vi "PhysMon-Options Dialog.vi"(0 "Options":T1={"Min Interval"=0.0, "HR from ABR?"=FALSE, "HR Scale"={"Slope"=0.0, "Offset"=0.0, "Limits"={"Min"=0.0, "Max"=0.0}, "term config"=-1}, "Temp Scale"={"Slope"=0.0, "Offset"=0.0, "Limits"={"Min"=0.0, "Max"=0.0}, "term config"=-1}, "Lock?"=FALSE, "Temp Sensor"=enum."YSI", "EKG"={"Sample duration (s)"=0.0}} {"Temp Scale"."term config" items=["default"=-1, "RSE"=10083, "NRSE"=10078, "Differential"=10106, "Pseudodifferential"=12529]; "HR Scale"."term config" items=["default"=-1, "RSE"=10083, "NRSE"=10078, "Differential"=10106, "Pseudodifferential"=12529]}) -> (4 "Options Out":T1={"Min Interval"=0.0, "HR from ABR?"=FALSE, "HR Scale"={"Slope"=0.0, "Offset"=0.0, "Limits"={"Min"=0.0, "Max"=0.0}, "term config"=-1}, "Temp Scale"={"Slope"=0.0, "Offset"=0.0, "Limits"={"Min"=0.0, "Max"=0.0}, "term config"=-1}, "Lock?"=FALSE, "Temp Sensor"=enum."YSI", "EKG"={"Sample duration (s)"=0.0}} {"Temp Scale"."term config" items=["default"=-1, "RSE"=10083, "NRSE"=10078, "Differential"=10106, "Pseudodifferential"=12529]; "HR Scale"."term config" items=["default"=-1, "RSE"=10083, "NRSE"=10078, "Differential"=10106, "Pseudodifferential"=12529]}, 8 "Canceled?":bool)   [LabVIEW 2020]
uses:
  Typedefs/PhysMon-Options.ctl
  Typedefs/PhysMon-Scale.ctl
  Typedefs/PhysMon-TempSensor.ctl
  Typedefs/PhysMon-HR From EKG Settings.ctl
panel:
  in  "HRTab":enum32{"Cardiotach", "EKG"}(tab)
  in  "HR Slope":dbl caption="Scale (bpm/V)"
  in  "HR Offset":dbl caption="Offset (bpm)"
  in  "Reset HR":bool
  in  "Test":bool
  in  "Sample size (s)":dbl
  in  "Sensor":enum16{"YSI", "FHC", "Custom"}(ring)
  in  "dummy":i32(ring)=10078 items=["default"=-1, "RSE"=10083, "NRSE"=10078, "Differential"=10106, "Pseudodifferential"=12529]
  in  "Calibrate":bool
  in  "TInputConfig":i32(ring) caption="Input configuration" items=["default"=-1, "RSE"=10083, "NRSE"=10078, "Differential"=10106, "Pseudodifferential"=12529]
  in  "Lock?":bool caption="Acquire vitals only when the system is idle"
  in  "HR from ABR":bool caption="Measure from raw EKG"
  in  "Reset Temp":bool
  in  "Temp Offset":dbl caption="Offset (deg C)"
  in  "Temp Slope":dbl caption="Scale (deg C/V)"
  in  "HR Max":dbl caption="Alarm max (bpm)"
  in  "HR Min":dbl caption="Alarm min (bpm)"
  in  "Min Interval":dbl caption="Minimum time between vital signs acquisition (min)"
  in  "Cancel":bool
  in  "OK":bool
  # "Heart Rate"
  # "Temperature"
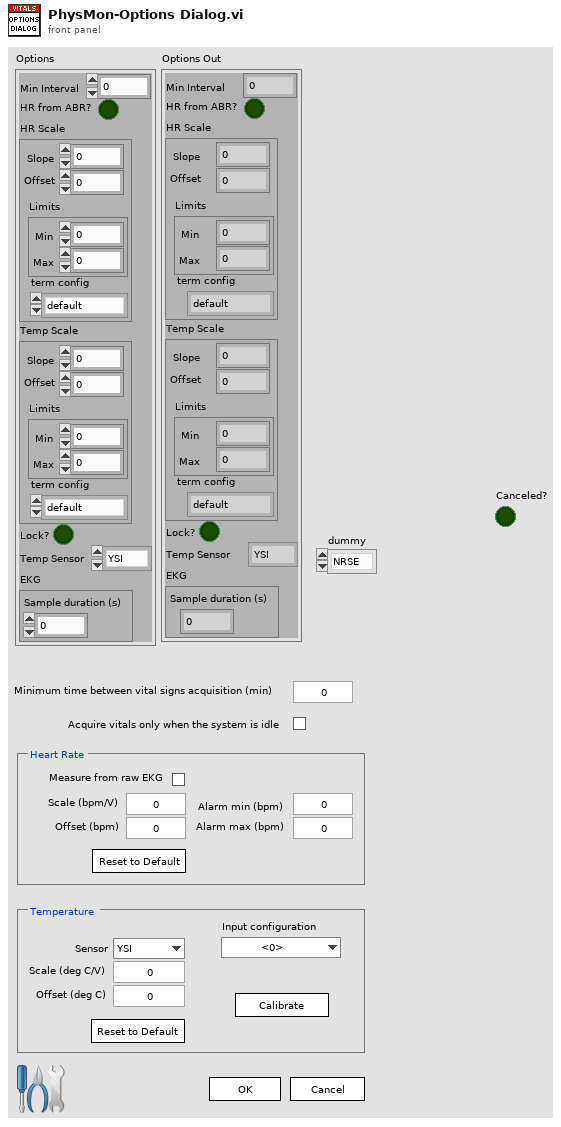
[diagram p1: front panel]
types:
  T1 = typedef "PhysMon-Options.ctl" = cluster{"Min Interval":dbl, "HR from ABR?":bool, "HR Scale":T2, "Temp Scale":T2, "Lock?":bool, "Temp Sensor":T3, "EKG":T4}
  T2 = typedef "PhysMon-Scale.ctl" = cluster{"Slope":dbl, "Offset":dbl, "Limits":cluster{"Min":dbl, "Max":dbl}, "term config":i32}
  T3 = typedef "PhysMon-TempSensor.ctl" = enum16{"YSI", "FHC", "Custom"}
  T4 = typedef "PhysMon-HR From EKG Settings.ctl" = cluster{"Sample duration (s)":dbl}
  T5 = enum8{"Enabled", "Disabled", "Disabled and Grayed Out"}
  T6 = typedef "LVStringsAndValuesArrayTypeDef_I32.ctl" = cluster{"String":string, "Value":i32}[]
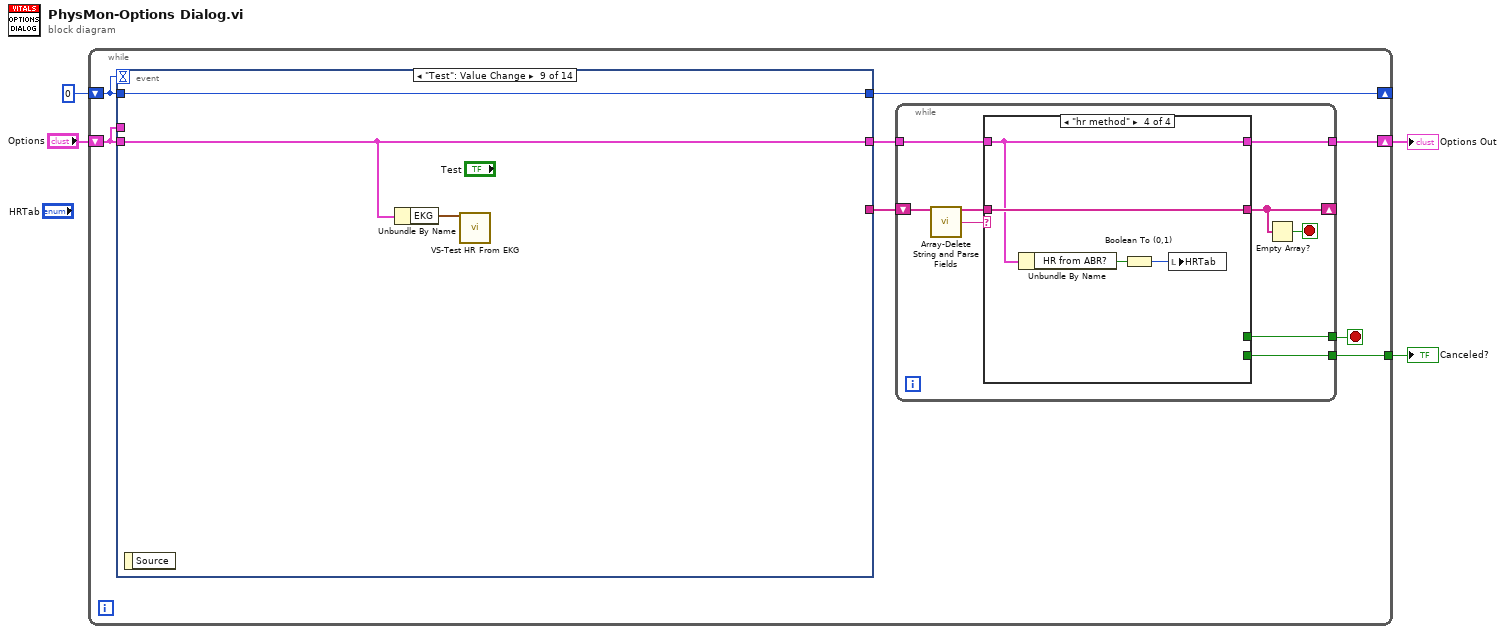
[diagram p0: block diagram]
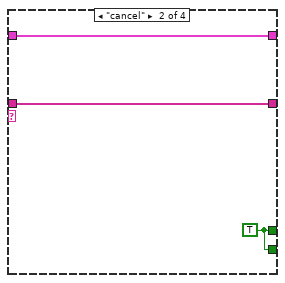
[diagram p3: hidden frame]
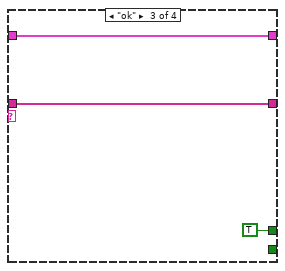
[diagram p4: hidden frame]
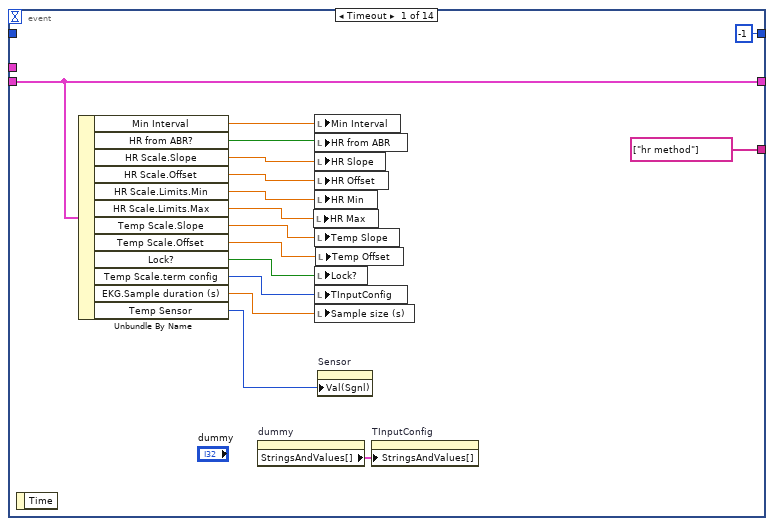
[diagram p5: hidden frame]
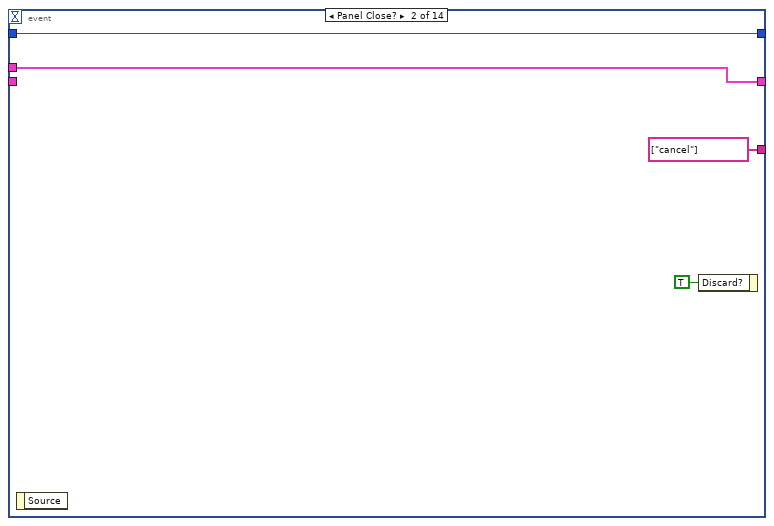
[diagram p6: hidden frame]
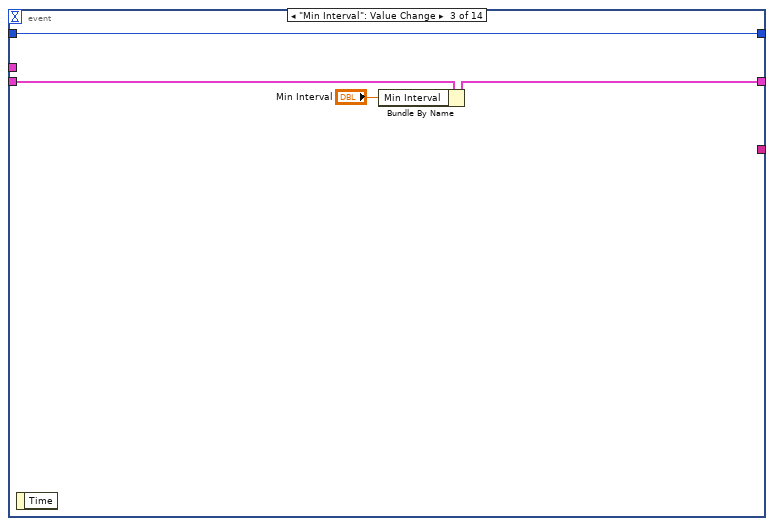
[diagram p7: hidden frame]
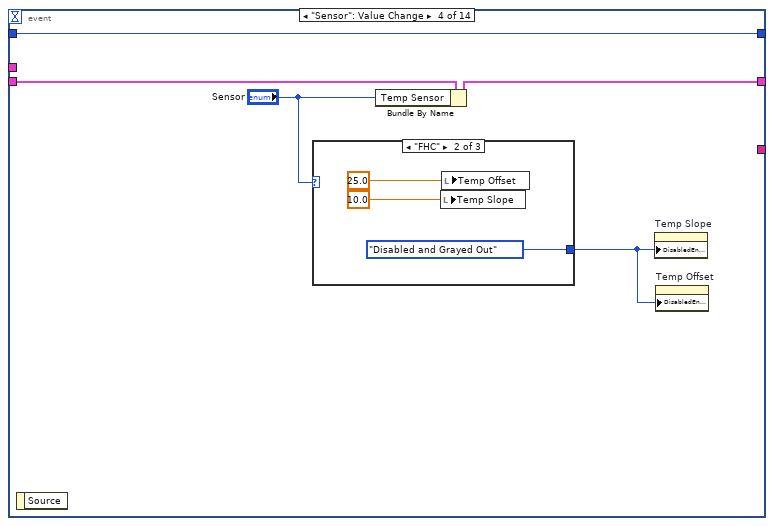
[diagram p8: hidden frame]
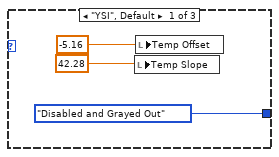
[diagram p9: hidden frame]
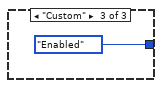
[diagram p10: hidden frame]
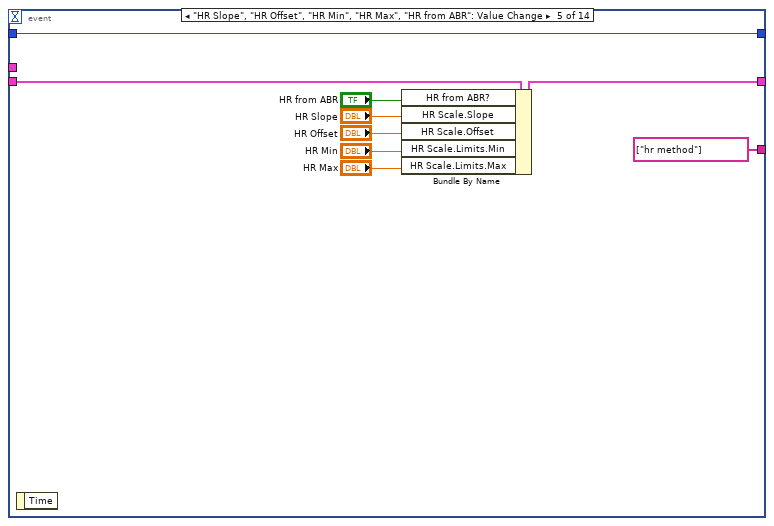
[diagram p11: hidden frame]
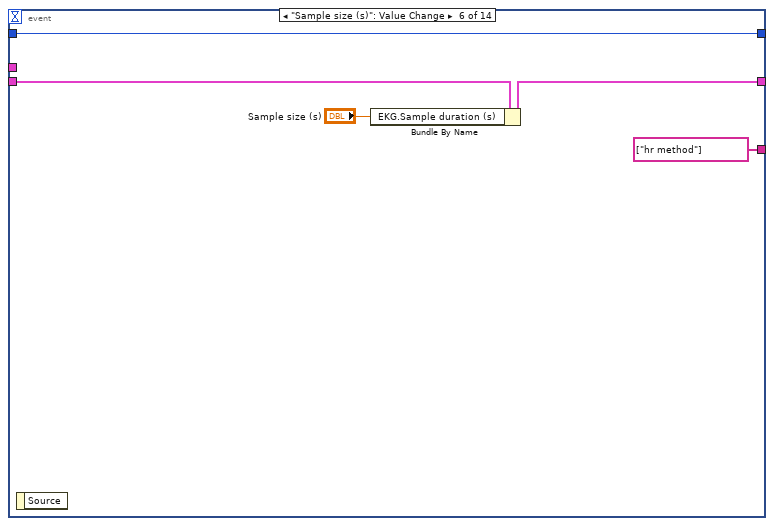
[diagram p12: hidden frame]
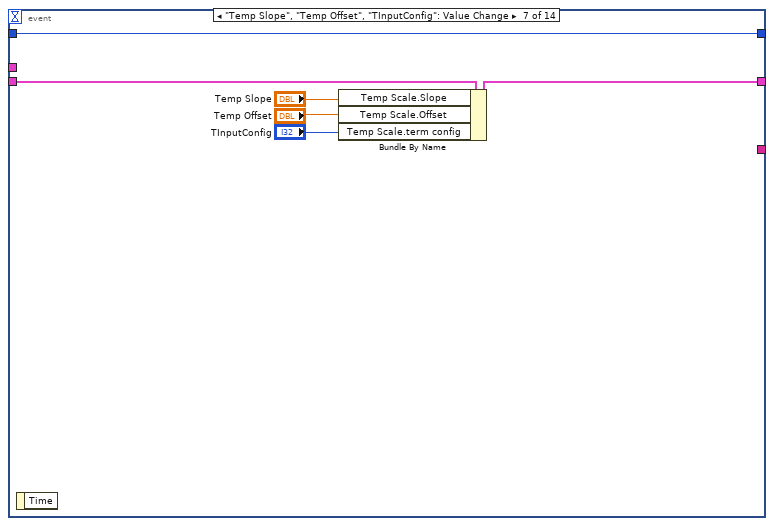
[diagram p13: hidden frame]
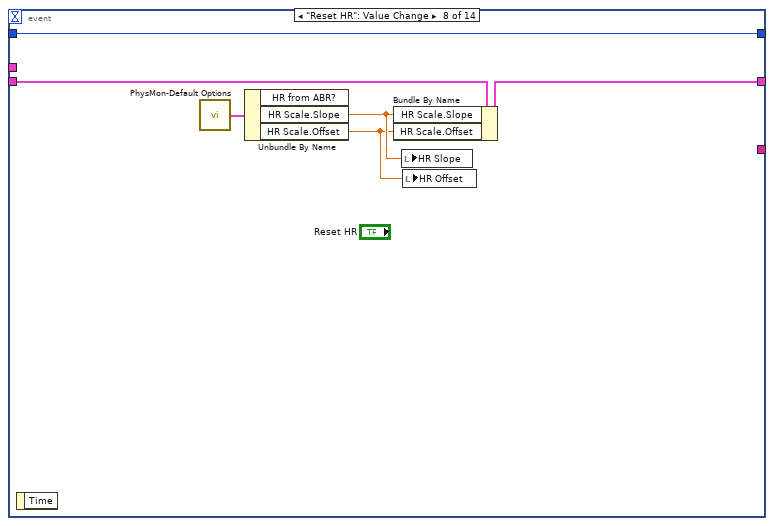
[diagram p14: hidden frame]
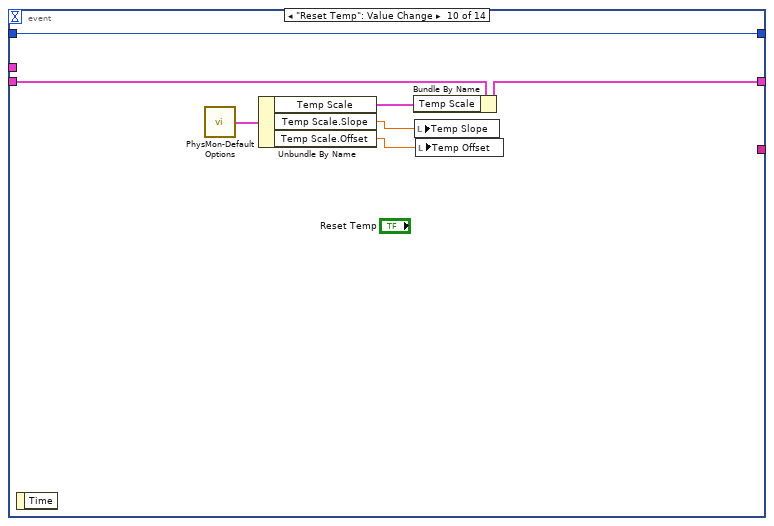
[diagram p15: hidden frame]
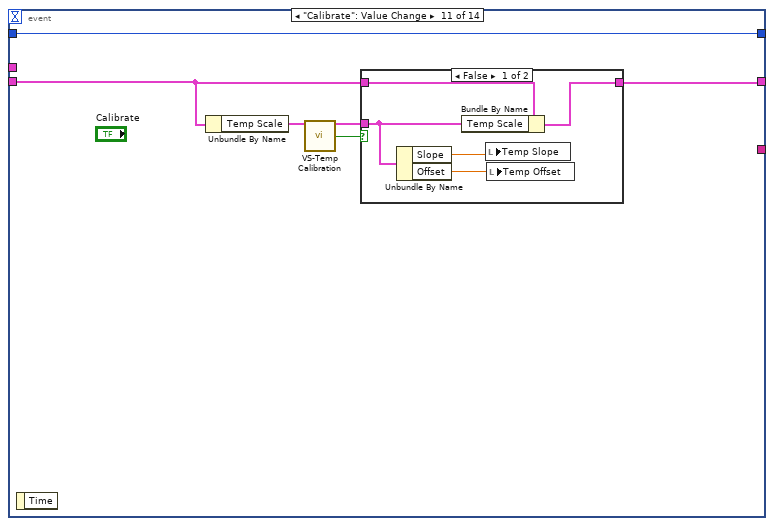
[diagram p16: hidden frame]
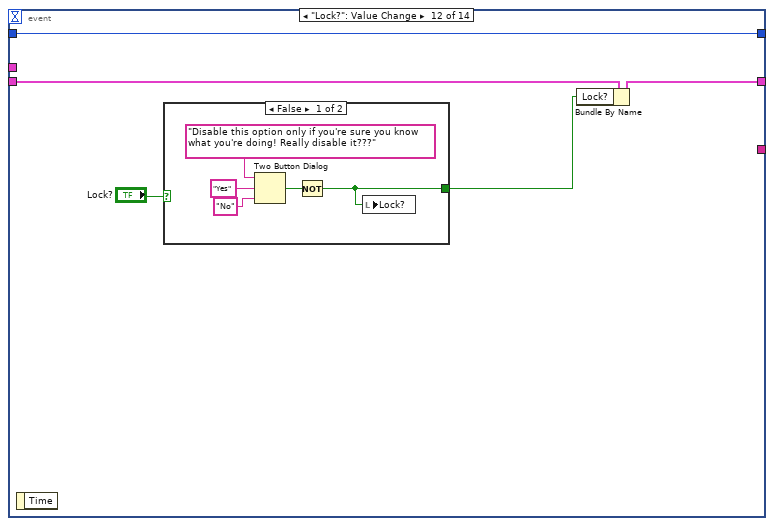
[diagram p18: hidden frame]
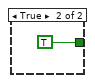
[diagram p19: hidden frame]
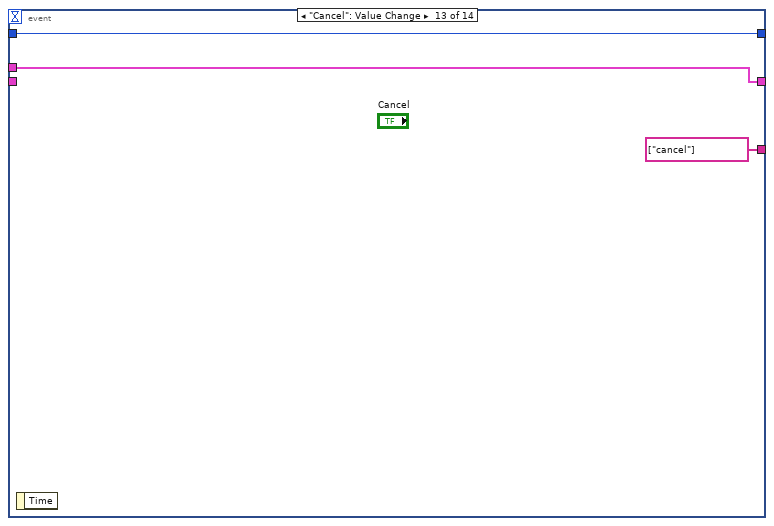
[diagram p20: hidden frame]
diagram:
  n1 = while {
    shift-right: [w12] -> _
    shift-left: 0 -> [w10]
    shift-right: [w9] -> w2
    shift-left: "Options" -> [w11]
    tunnel: [w5] -> w1
    stop <- w6 stop-if-true
    n2 = event shown="[8] \"Test\": Value Change" {
      selector: _ -> [_ _ _ _ _ _ _ _ _ _ _ _ _ _]
      dyn-events: _ -> [_ _ _ _ _ _ _ _ _ _ _ _ _ _]
      timeout: w10 -> [_ _ _ _ _ _ _ _ _ _ _ _ _ _]
      tunnel: [-1 w52 w54 w58 w71 w81 w84 w90 w98 w99 w106 w118 w130 w133] -> w12
      tunnel: w11 -> [w48 _ w57 w62 w78 w83 w89 w95 w97 w105 w109 w122 _ w134]
      tunnel: [w48 w50 w56 w61 w77 w82 w88 w93 w97 w104 w108 w120 w131 w134] -> w8
      tunnel: w11 -> [_ w50 _ _ _ _ _ _ _ _ _ _ w131 _]
      tunnel: w10 -> [_ w52 w54 w58 w71 w81 w84 w90 w98 w99 w106 w118 w130 w133]
      tunnel: [string[] ["hr method"] string[] ["cancel"] _ _ string[] ["hr method"] string[] ["hr method"] _ _ _ _ _ _ string[] ["cancel"] string[] ["ok"]] -> w7
      event Timeout {
        n3 = event-data() -> ()  [unwired: 1 in, 1 out]
        n4 = Unbundle By Name(w48) -> ("Min Interval"=w47:dbl, "HR from ABR?"=w46:bool, "HR Scale.Slope"=w45:dbl, "HR Scale.Offset"=w44:dbl, "HR Scale.Limits.Min"=w43:dbl, "HR Scale.Limits.Max"=w42:dbl, "Temp Scale.Slope"=w41:dbl, "Temp Scale.Offset"=w40:dbl, "Lock?"=w39:bool, "Temp Scale.term config"=w38:i32, "EKG.Sample duration (s)"=w34:dbl, "Temp Sensor"=w36:T3)
        n5 = property on="dummy" class="Ring (strict)"() -> ("StringsAndValues[]"=w37:T6)  [unwired: 2 in, 2 out]
        n6 = local write "HR Max"(w42) -> ()
        n7 = local write "Min Interval"(w47) -> ()
        n8 = local write "HR from ABR"(w46) -> ()
        n9 = local write "HR Slope"(w45) -> ()
        n10 = local write "HR Offset"(w44) -> ()
        n11 = local write "HR Min"(w43) -> ()
        n12 = local write "Temp Slope"(w41) -> ()
        n13 = local write "Lock?"(w39) -> ()
        n14 = local write "TInputConfig"(w38) -> ()
        n15 = local write "Sample size (s)"(w34) -> ()
        n16 = local write "Temp Offset"(w40) -> ()
        n17 = property on="Sensor" class="Enum (strict)"("Val(Sgnl)"=w36) -> ()  [unwired: 2 in, 2 out]
        n18 = property on="TInputConfig" class="Ring (strict)"("StringsAndValues[]"=w37) -> ()  [unwired: 2 in, 2 out]
      }
      event Panel Close? {
        n19 = event-data() -> ()  [unwired: 1 in, 1 out]
        n20 = event-data("Discard?"=TRUE) -> ()  [unwired: 1 in, 1 out]
      }
      event "Min Interval": Value Change {
        n21 = event-data() -> ()  [unwired: 1 in, 1 out]
        n22 = Bundle By Name(cluster=w57, "Min Interval"="Min Interval") -> (w56:T1)
      }
      event "Sensor": Value Change {
        n23 = event-data() -> ()  [unwired: 1 in, 1 out]
        n24 = case shown="\"FHC\"" "Sensor" {
          tunnel: [T5."Disabled and Grayed Out" ("Disabled") T5."Disabled and Grayed Out" ("Disabled") T5."Enabled" ("Disabled")] -> w59
          frame "YSI", Default {
            n25 = local write "Temp Slope"(42.28 ("y")) -> ()
            n26 = local write "Temp Offset"(-5.16 ("y")) -> ()
          }
          frame "FHC" {
            n27 = local write "Temp Slope"(10.0 ("y")) -> ()
            n28 = local write "Temp Offset"(25.0 ("y")) -> ()
          }
          frame "Custom" {
          }
        }
        n29 = Bundle By Name(cluster=w62, "Temp Sensor"="Sensor") -> (w61:T1)
        n30 = property on="Temp Slope" class="DigNum (strict)"("DisabledEnum"=w59) -> ()  [unwired: 2 in, 2 out]
        n31 = property on="Temp Offset" class="DigNum (strict)"("DisabledEnum"=w59) -> ()  [unwired: 2 in, 2 out]
      }
      event "HR Slope", "HR Offset", "HR Min", "HR Max", "HR from ABR": Value Change {
        n32 = event-data() -> ()  [unwired: 1 in, 1 out]
        n33 = Bundle By Name(cluster=w78, "HR from ABR?"="HR from ABR", "HR Scale.Slope"="HR Slope", "HR Scale.Offset"="HR Offset", "HR Scale.Limits.Min"="HR Min", "HR Scale.Limits.Max"="HR Max") -> (w77:T1)
      }
      event "Sample size (s)": Value Change {
        n34 = event-data() -> ()  [unwired: 1 in, 1 out]
        n35 = Bundle By Name(cluster=w83, "EKG.Sample duration (s)"="Sample size (s)") -> (w82:T1)
      }
      event "Temp Slope", "Temp Offset", "TInputConfig": Value Change {
        n36 = event-data() -> ()  [unwired: 1 in, 1 out]
        n37 = Bundle By Name(cluster=w89, "Temp Scale.Slope"="Temp Slope", "Temp Scale.Offset"="Temp Offset", "Temp Scale.term config"="TInputConfig") -> (w88:T1)
      }
      event "Reset HR": Value Change {
        n38 = event-data() -> ()  [unwired: 1 in, 1 out]
        n39 = call "PhysMon-Default Options.vi"() -> ("Options"=w94:T1)  [unwired: 14 in, 1 out]
        n40 = Unbundle By Name(w94) -> ("HR Scale.Slope"=w92:dbl, "HR Scale.Offset"=w91:dbl)  [unwired: 1 out]
        n41 = Bundle By Name(cluster=w95, "HR Scale.Slope"=w92, "HR Scale.Offset"=w91) -> (w93:T1)
        n42 = local write "HR Slope"(w92) -> ()
        n43 = local write "HR Offset"(w91) -> ()
      }
      event "Test": Value Change {
        n44 = event-data() -> ()  [unwired: 1 in, 1 out]
        n45 = Unbundle By Name(w97) -> ("EKG"=w96:T4)
        n46 = call "VS-Test HR From EKG.vi"("Cluster In"=w96) -> ()  [unwired: 14 in, 1 out]
      }
      event "Reset Temp": Value Change {
        n47 = event-data() -> ()  [unwired: 1 in, 1 out]
        n48 = call "PhysMon-Default Options.vi"() -> ("Options"=w103:T1)  [unwired: 14 in, 1 out]
        n49 = Unbundle By Name(w103) -> ("Temp Scale"=w102:T2, "Temp Scale.Slope"=w101:dbl, "Temp Scale.Offset"=w100:dbl)
        n50 = Bundle By Name(cluster=w105, "Temp Scale"=w102) -> (w104:T1)
        n51 = local write "Temp Slope"(w101) -> ()
        n52 = local write "Temp Offset"(w100) -> ()
      }
      event "Calibrate": Value Change {
        n53 = event-data() -> ()  [unwired: 1 in, 1 out]
        n54 = Unbundle By Name(w109) -> ("Temp Scale"=w111:T2)
        n55 = call "VS-Temp Calibration.vi"("Scale"=w111) -> ("Cluster out"=w107:T2, "Canceled?"=w110:bool)  [unwired: 13 in]
        n56 = case shown="False" w110 {
          tunnel: w109 -> [w116 w117]
          tunnel: [w115 w117] -> w108
          tunnel: w107 -> [w114 _]
          frame False {
            n57 = Unbundle By Name(w114) -> ("Slope"=w112:dbl, "Offset"=w113:dbl)
            n58 = Bundle By Name(cluster=w116, "Temp Scale"=w114) -> (w115:T1)
            n59 = local write "Temp Slope"(w112) -> ()
            n60 = local write "Temp Offset"(w113) -> ()
          }
          frame True {
          }
        }
      }
      event "Lock?": Value Change {
        n61 = event-data() -> ()  [unwired: 1 in, 1 out]
        n62 = case shown="False" "Lock?" {
          tunnel: [w123 TRUE] -> w119
          frame False {
            n63 = Two Button Dialog(message="Disable this option only if you're sure you know what you're doing! Really disable it???", 1:"No" ("F button name (\"Cancel\")"), 2:"Yes" ("T button name (\"OK\")")) -> (T button?=w124:bool)
            n64 = Not(x=w124) -> (.not. x?=w123:bool)
            n65 = local write "Lock?"(w123) -> ()
          }
          frame True {
          }
        }
        n66 = Bundle By Name(cluster=w122, "Lock?"=w119) -> (w120:T1)
      }
      event "Cancel": Value Change {
        n67 = event-data() -> ()  [unwired: 1 in, 1 out]
      }
      event "OK": Value Change {
        n68 = event-data() -> ()  [unwired: 1 in, 1 out]
      }
    }
    n69 = while {
      shift-right: [w21] -> _
      shift-left: w7 -> [w18]
      tunnel: [w19] -> w6
      tunnel: [w15] -> w9
      tunnel: w8 -> [w14]
      tunnel: [w13] -> w5
      stop <- w20 stop-if-true
      n70 = call "Array-Delete String and Parse Fields.vi"("Array in"=w18) -> ("Array out"=w17:string[], "Field 1"=w16:string)  [unwired: 10 in, 3 out]
      n71 = case shown="\"hr method\"" w16 {
        tunnel: w17 -> [w23 w26 w29 w33]
        tunnel: [w23 w26 w29 w33] -> w21
        tunnel: [_ w24 TRUE _] -> w19
        tunnel: [w22 w25 w28 w32] -> w15
        tunnel: w14 -> [w22 w25 w28 w32]
        tunnel: [_ w24 _ _] -> w13
        frame "", Default {
        }
        frame "cancel" {
          w24 = TRUE
        }
        frame "ok" {
        }
        frame "hr method" {
          n72 = Unbundle By Name(w32) -> ("HR from ABR?"=w31:bool)
          n73 = Boolean To (0,1)(Boolean=w31) -> (0, 1=w30:i16)
          n74 = local write "HRTab"(w30) -> ()
        }
      }
      n75 = Empty Array?(array=w21) -> (empty?=w20:bool)
    }
  }
  "Options Out" <- w2
  "Canceled?" <- w1
